vi "NiFpga_HdlRegister_WriteU32.vi"(6 "Enable Error Checking":bool=TRUE, 7 "error in (no error)":errorcluster, 8 "Value":u32, 9 "Offset":u32, 10 "FPGA VI Reference In":refnum<k20>) -> (0 "error out":errorcluster, 3 "FPGA VI Reference Out":refnum<k20>)   [LabVIEW 2023]
doc: "Dynamically reads the register at the provided offset. Set check for errors to true to check for errors such as if the register offset is invalid or if the register is running in an external clock domain that might not be running."
uses:
  NiFpga.dll
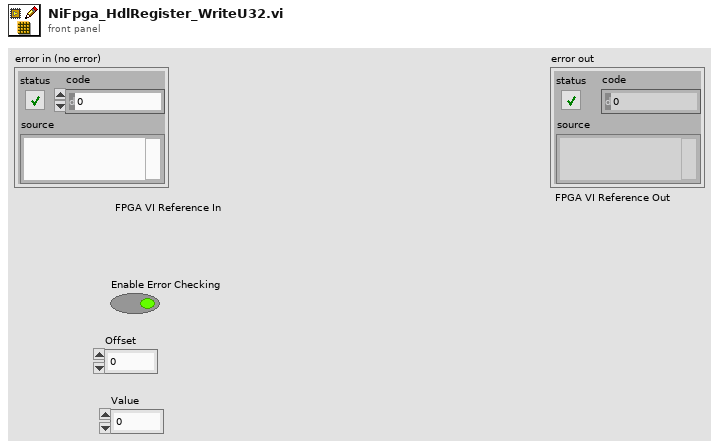
[diagram p1: front panel]
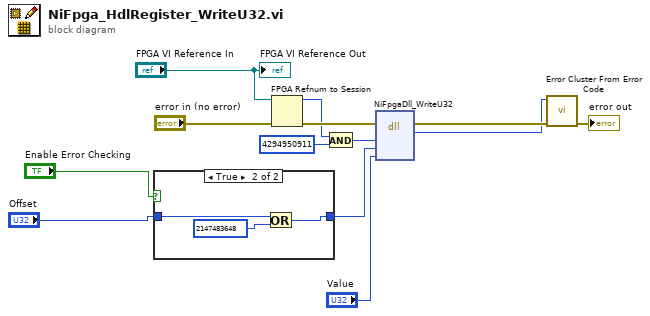
[diagram p0: block diagram]
diagram:
  n1 = case shown="True" "Enable Error Checking" {
    tunnel: "Offset" -> [w14 w17]
    tunnel: [w14 w15] -> w6
    frame False {
    }
    frame True {
      n2 = Or(x=w17, y=u32 2147483648) -> (x .or. y?=w15:u32)
    }
  }
  n3 = FPGA Refnum to Session(4:"error in (no error)", 7:"FPGA VI Reference In") -> (0:w11:errorcluster, 3:w4:u64)
  n4 = And(x=w4, y=u64 4294950911) -> (x .and. y?=w2:u64)
  n5 = dll-call lib="NiFpga.*" fn="NiFpgaDll_WriteU32"(error in=w11, "session"=w2, "offset"=w6, "value"="Value") -> (error out=w9:errorcluster, "return type"=w8:i32)  [unwired: 5 in, 1 out]
  n6 = call <vilib>:"Error Cluster From Error Code.vi"("error in (no error)"=w9, "error code (0)"=w8) -> ("error out"=→"error out":errorcluster)  [unwired: 7 in]
  "FPGA VI Reference Out" <- "FPGA VI Reference In"
